vi "Large Number Operation.Async.vi"(10 "Parameters":variant, 11 "Process":refnum<class "Process.lvclass">) -> ()   [LabVIEW 2021, in "Large Number Operation Engine.lvlib"]
uses:
  Large Number Operation Engine.lvlib
  <vilib>/NI/NIVS Inline Async API/_VS Inline Async API/Process/Process.lvclass
  <vilib>/gRPC/LabVIEW gRPC Library/Shared/grpcId.ctl
  Shared/Compiled.Settings.ctl
  <vilib>/NI/NIVS Inline Async API/_VS Inline Async API/Process/Process.lvclass/Process.ctl
  labview-grpc-source/veristand-grpc_client/RPC Messages/veristand_Request.ctl
  <vilib>/NI/NIVS Inline Async API/_Data Access Engine/Access Type Classes/Read/Read.lvclass/Read.ctl
  <vilib>/NI/NIVS Inline Async API/_Data Access Engine/Access Type Classes/Write/Write.lvclass/Write.ctl
  <vilib>/NI/NIVS Inline Async API/_Data Access Engine/Data Access Engine/Methods/Read.Data.vi
  <vilib>/NI/NIVS Inline Async API/_Data Access Engine/Data Access Engine/Methods/Write.Data.vi
  <vilib>/NI/NIVS Inline Async API/_VS Inline Async API/Process/Data Member Access/Read Data Access.vi
  <vilib>/NI/NIVS Inline Async API/_VS Inline Async API/Error Handling Process/SubVIs/Error.ConvertArray.vi
  <vilib>/NI/NIVS Inline Async API/_Data Access Engine/Access Type Classes/Read/Read.ProcessData.vi
  <vilib>/NI/NIVS Inline Async API/_Data Access Engine/Access Type Classes/Write/Write.ProcessData.vi
  <vilib>/NI/NIVS Inline Async API/_Data Access Engine/Access Type Classes/Write/Write.Buffer.vi
  <vilib>/NI/NIVS Inline Async API/_Data Access Engine/Access Type Classes/Write/Write.Commit.vi
  <vilib>/NI/NIVS Inline Async API/_Data Access Engine/Data Access Engine/Methods/Write.Lookup.vi
  <vilib>/NI/NIVS Inline Async API/_Data Access Engine/Data Access Engine/Methods/Read.Lookup.vi
  <vilib>/NI/NIVS Inline Async API/_Data Access Engine/Data Access Engine/Data Access Engine.lvclass
  labview-grpc-source/veristand-grpc_client/VeriStandgrpc_client.lvlib
  Shared/Large Number Operation Shared.lvlib
  <vilib>/gRPC/LabVIEW gRPC Library/grpc-lvsupport-release.lvlib
panel:
  out "gRPC ID Out":T1
  out "Sum":string
  out "Numbers":string[](array[string])
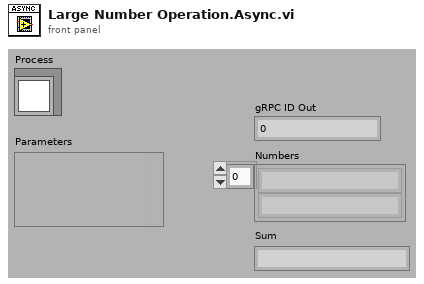
[diagram p1: front panel]
types:
  T1 = typedef "grpc-lvsupport-release.lvlib/grpcId.ctl" = u64
  T2 = typedef "Large Number Operation Shared.lvlib/Compiled.Settings.ctl" = cluster{"Name":string, "Async Init Timeout":u16, "Address":string}
  T3 = enum32{"Invalid", "Standard", "Closed", "Hidden", "Minimized", "Maximized"}
  T4 = typedef "Data Access Engine.lvlib/Data Access Engine.lvclass/Write.DVR.ctl" = refnum<data-value>
  T5 = typedef "Data Access Engine.lvlib/Data Access Engine.lvclass/Read.DVR.ctl" = refnum<data-value>
  T6 = typedef "VeriStandgrpc_client.lvlib/veristand_Request.ctl" = cluster{"server":string, "channel":string, "data":string}
  T7 = typedef "VeriStandgrpc_client.lvlib/veristand_Reponse.ctl" = cluster{"status":string, "data":string}
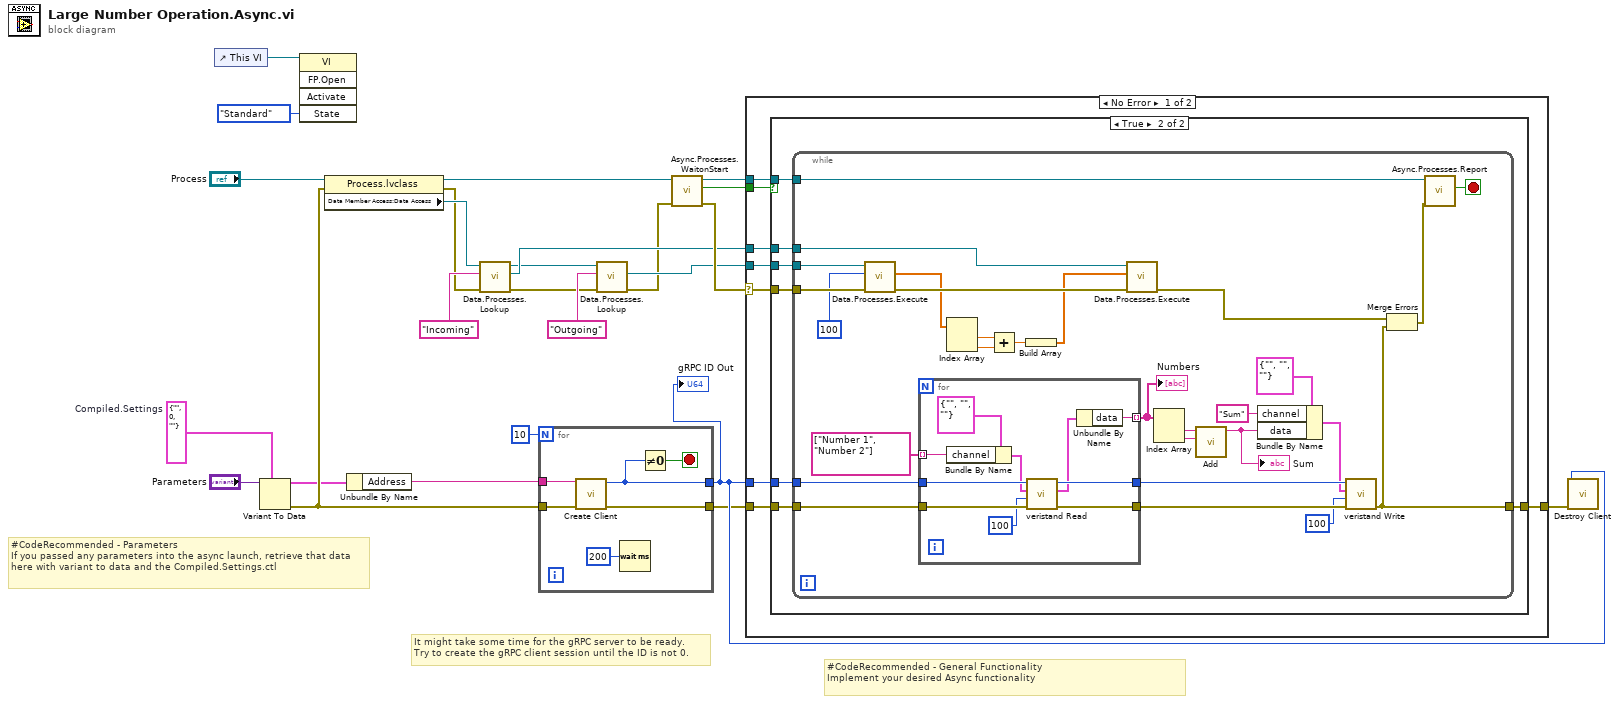
[diagram p0: block diagram]
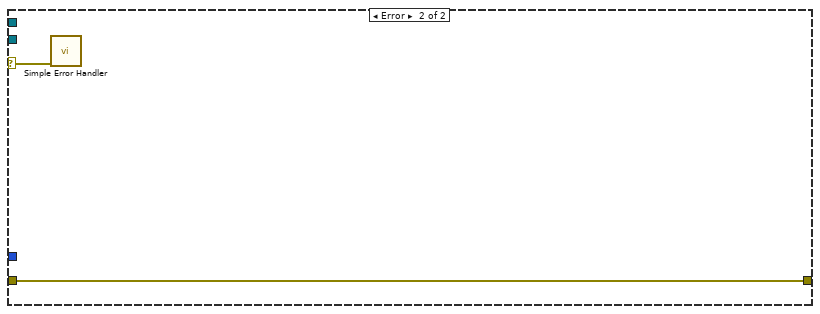
[diagram p3: hidden frame]
diagram:
  w3 = T2 {"Name"="", "Async Init Timeout"=0, "Address"=""}  # Compiled.Settings
  # "It might take some time for the gRPC server to be ready.\nTry to create the gRPC client session until the ID is not 0."
  # "#CodeRecommended - General Functionality\nImplement your desired Async functionality"
  # "#CodeRecommended - Parameters\nIf you passed any parameters into the async launch, retrieve that data here with variant to data and the Compiled.Settings.ctl"
  n1 = control-ref of="This VI"() -> (w5:refnum<vi>)
  n2 = Variant To Data(type=w3, Variant="Parameters") -> (data=w2:T2, error out=w10:errorcluster)  [unwired: 1 in]
  n3 = invoke class="VI" method="FP.Open"(reference=w5, "State"=T3."Standard") -> ()  [unwired: 3 in, 5 out]
  n4 = property class="Process.lvclass"(reference="Process", error in=w10) -> (reference out=w14:refnum<class "Process.lvclass">, error out=w12:errorcluster, "Data Member Access:Data Access"=w13:refnum<class "Data Access Engine.lvclass">)
  n5 = Unbundle By Name(w2) -> ("Address"=w1:string)
  n6 = call-poly <vilib>:"Data.Processes.Lookup.vi"("error in (no error)"=w12, "Name"="Incoming", "Data Access API in"=w13) -> ("error out"=w19:errorcluster, "Ref"=w18:T4, "Data Access API out"=w17:refnum<class "Data Access Engine.lvclass">)  [unwired: 5 in, 1 out]
  n7 = for {
    N: 10 -> [_]
    tunnel: w10 -> [w31]
    tunnel: [w28] -> w8
    tunnel: [w29] -> w7
    tunnel: w1 -> [w26]
    stop <- w27 stop-if-true
    n8 = call "Create Client.vi"("error in"=w31, "address"=w26) -> ("error out"=w29:errorcluster, "gRPC ID Out"=w28:T1)  [unwired: 8 in]
    n9 = Wait (ms)(milliseconds to wait=u32 200) -> ()  [unwired: 1 out]
    n10 = Not Equal To 0?(x=w28) -> (x != 0?=w27:bool)
  }
  "gRPC ID Out" <- w8
  n11 = call-poly <vilib>:"Data.Processes.Lookup.vi"("error in (no error)"=w19, "Name"="Outgoing", "Data Access API in"=w17) -> ("error out"=w16:errorcluster, "Ref"=w21:T5)  [unwired: 5 in, 2 out]
  n12 = call <vilib>:"Async.Processes.WaitonStart.vi"("error in (no error)"=w16, "Process"=w14) -> ("error out"=w23:errorcluster, "Execute"=w25:bool, "Process out"=w24:refnum<class "Process.lvclass">)  [unwired: 7 in]
  n13 = case shown="No Error" w23 {
    selector: w23 -> [w35 w87]
    tunnel: w25 -> [w39 _]
    tunnel: w24 -> [w38 _]
    tunnel: w18 -> [w37 _]
    tunnel: w21 -> [w36 _]
    tunnel: w8 -> [w34 _]
    tunnel: w7 -> [w33 w86]
    tunnel: [w32 w86] -> w6
    frame No Error {
      n14 = case shown="True" w39 {
        tunnel: w35 -> [_ w44]
        tunnel: w38 -> [_ w45]
        tunnel: w36 -> [_ w47]
        tunnel: w37 -> [_ w46]
        tunnel: w34 -> [_ w43]
        tunnel: w33 -> [w40 w42]
        tunnel: [w40 w41] -> w32
        frame False {
        }
        frame True {
          n15 = while {
            tunnel: w44 -> [w71]
            tunnel: w45 -> [w75]
            tunnel: w47 -> [w73]
            tunnel: w46 -> [w72]
            tunnel: w43 -> [w61]
            tunnel: w42 -> [w59]
            tunnel: [w48] -> w41
            stop <- w74 stop-if-true
            n16 = call-poly <vilib>:"Data.Processes.Execute.vi"("error in (no error)"=w71, "timeout ms"=100, "Ref"=w73) -> ("error out"=w69:errorcluster, "Values"=w68:dbl[])  [unwired: 6 in, 1 out]
            n17 = for {
              tunnel: w61 -> [w85]
              tunnel: string[] ["Number 1", "Number 2"] -> [w83] mode=indexing
              tunnel: w59 -> [w81]
              tunnel: [w79] -> w55
              tunnel: [w78] -> w54
              tunnel: [w76] -> w58 mode=indexing
              n18 = Bundle By Name(cluster=T6 {"server"="", "channel"="", "data"=""} ("Request Data"), "channel"=w83) -> (w82:T6)
              n19 = call "veristand Read.vi"("error in"=w81, "timeout (ms)"=100, "Request Data"=w82, "gRPC ID"=w85) -> ("error out"=w78:errorcluster, "Response Data"=w77:T7, "gRPC ID out"=w79:T1)  [unwired: 5 in]
              n20 = Unbundle By Name(w77) -> ("data"=w76:string)
            }
            "Numbers" <- w58
            n21 = Index Array(array=w68) -> (element #1=w66:dbl, element #2=w67:dbl)  [unwired: 2 in]
            n22 = Add(x=w66, y=w67) -> (x+y=w65:dbl)
            n23 = Build Array(w65) -> (w64:dbl[])
            n24 = call-poly <vilib>:"Data.Processes.Execute.vi"("error in (no error)"=w69, "Values"=w64, "Ref"=w72) -> ("error out"=w63:errorcluster)  [unwired: 8 in]
            n25 = Index Array(array=w58) -> (element #1=w57:string, element #2=w56:string)  [unwired: 2 in]
            n26 = call "Add.vi"("Y"=w56, "X"=w57) -> ("Sum"=w51:string)  [unwired: 9 in]
            "Sum" <- w51
            n27 = Bundle By Name(cluster=T6 {"server"="", "channel"="", "data"=""} ("Request Data"), "channel"="Sum", "data"=w51) -> (w50:T6)
            n28 = call "veristand Write.vi"("error in"=w54, "timeout (ms)"=100, "Request Data"=w50, "gRPC ID"=w55) -> ("error out"=w48:errorcluster)  [unwired: 5 in, 2 out]
            n29 = Merge Errors(w63, w48) -> (w62:errorcluster)
            n30 = call <vilib>:"Async.Processes.Report.vi"("Error"=w62, "Process in"=w75) -> ("Stop"=w74:bool)  [unwired: 8 in, 1 out]
          }
        }
      }
    }
    frame Error {
      n31 = call <vilib>:"Simple Error Handler.vi"("error in (no error)"=w87) -> ()  [unwired: 4 in, 5 out]
    }
  }
  n32 = call "Destroy Client.vi"("error in"=w6, "gRPC ID"=w8) -> ()  [unwired: 9 in, 1 out]
